vi "sendSubDataCommunication.vi"(6 "newValue (T)":bool=TRUE, 8 "error in (no error)":errorcluster, 9 "value":variant, 10 "subDataSV":T1, 11 "Cmtr in":refnum<class "Communicator.lvclass">) -> (0 "error out":errorcluster, 3 "Cmtr out":refnum<class "Communicator.lvclass">)   [LabVIEW 2015, in "EXACommunications.lvlib" / "Communicator.lvclass"]
doc: "Writes value to SubData SV."
uses:
  Communicator.lvclass
  Typedefs/SubDataSV.ctl
  ComponentTemplateCore/ComponentModel/ComponentModel/Typedefs/CommunicationConfig.ctl
  ComponentTemplateCore/ComponentModel/ComponentModel/SVMessenger/SVMessenger.lvclass
  ComponentTemplateCore/ComponentModel/ComponentModel/Messenger/Messenger.lvclass/Messenger.ctl
  ComponentTemplateCore/ComponentModel/ComponentModel/Messenger/Messenger.lvclass
  Typedefs/EXATypedefs.lvlib
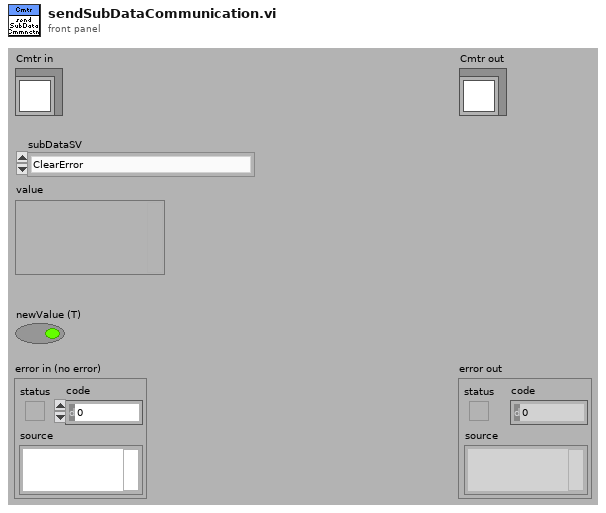
[diagram p1: front panel]
types:
  T1 = typedef "EXATypedefs.lvlib/SubDataSV.ctl" = enum16{"ClearError", "Disable", "Enable", "Exit", "GoToStandby", "HeartbeatIn", "Start"}
  T2 = typedef "CommunicationConfig.ctl" = cluster{"hostComputerAddress":string, "ComponentAcronym":string, "InstanceIdentifier":i32}
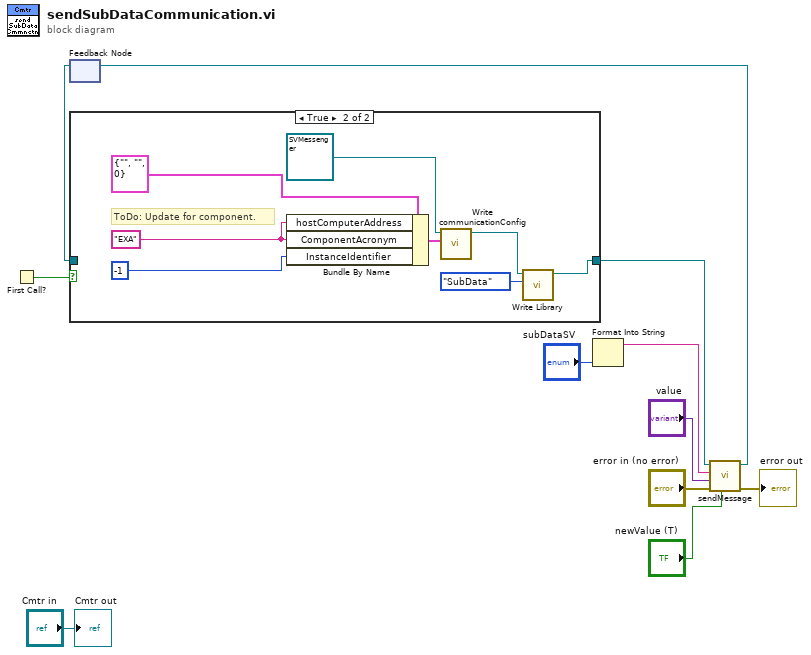
[diagram p0: block diagram]
diagram:
  n1 = First Call?() -> (First Call?: T/F=w4:bool)
  n2 = feedback #1() -> (w2:refnum<class "SVMessenger.lvclass">)  [unwired: 1 in]
  n3 = case shown="True" w4 {
    tunnel: [w12 w13] -> w3
    tunnel: w2 -> [w12 _]
    frame False {
    }
    frame True {
      w19 = "EXA" ("hostComputerAddress")
      # "ToDo: Update for component."
      n4 = Bundle By Name(cluster=T2 {"hostComputerAddress"="", "ComponentAcronym"="", "InstanceIdentifier"=0} ("sharedVariableLibrariesConfig"), "hostComputerAddress"=w19, "ComponentAcronym"=w19, "InstanceIdentifier"=-1) -> (w17:T2)
      n5 = call "Write communicationConfig.vi"("communicationConfig"=w17, "Messenger in"=refnum<class "SVMessenger.lvclass"> refnum ("SVMessenger.lvclass")) -> ("Messenger out"=w15:refnum<class "SVMessenger.lvclass">)  [unwired: 9 in]
      n6 = call "Write Library.vi"("Library"=enum16{"PubData", "SubData"}."SubData", "Messenger in"=w15) -> ("Messenger out"=w13:refnum<class "SVMessenger.lvclass">)  [unwired: 9 in]
    }
  }
  n7 = Format Into String("subDataSV") -> (resulting string=w6:string)  [unwired: 3 in, 1 out]
  n8 = call "sendMessage.vi"("newValue (T)"="newValue (T)", "error in (no error)"="error in (no error)", "value"="value", "signalName"=w6, "Messenger in"=w3) -> ("error out"=→"error out":errorcluster, "Messenger out"=w5:refnum<class "SVMessenger.lvclass">)  [unwired: 5 in]
  n9 = feedback-in #1(w5) -> ()
  "Cmtr out" <- "Cmtr in"
